vi "Launcher.vi"(8 "Globals":refnum<data-value>, 9 "E-Stop":refnum<user-event>, 10 "Response":refnum<user-event>, 11 "RequestMQ":refnum<queue>) -> ()   [LabVIEW 2020, in "Module.lvlib" / "Module.lvclass"]
doc: "This template is for the Queued Message Handler design pattern.\n\nThe Event Handling Loop generates messages based on user interface actions.\n\nThe Message Handling Loop processes messages generated by the Event Handling Loop, or by other messages. The messages are string values, so new messages can be added easily to the Message Cases case structure in the Message Handling Loop. Each message cluster can also provide an optional value for Message Data, which is a variant that can be converted to whatever message-specific data is required."
uses:
  Module.lvclass
  RPC/TypeDefs/Request.ctl
  RPC/TypeDefs/Response.ctl
  Module.lvclass/Module.ctl
  <vilib>/ErrorRing/Error Ring.xnode
  RPC.lvlib
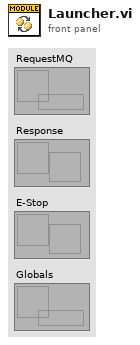
[diagram p1: front panel]
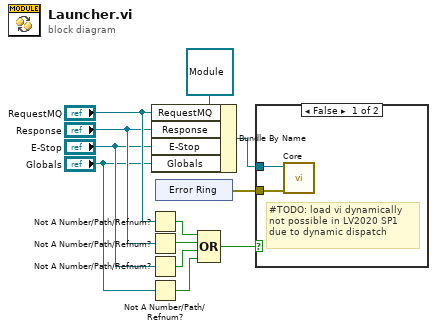
[diagram p0: block diagram]
diagram:
  n1 = Not A Number/Path/Refnum?(number/path/refnum="RequestMQ") -> (NaN/Path/Refnum?=w6:bool)
  n2 = Not A Number/Path/Refnum?(number/path/refnum="Response") -> (NaN/Path/Refnum?=w5:bool)
  n3 = Not A Number/Path/Refnum?(number/path/refnum="E-Stop") -> (NaN/Path/Refnum?=w4:bool)
  n4 = Not A Number/Path/Refnum?(number/path/refnum="Globals") -> (NaN/Path/Refnum?=w1:bool)
  n5 = Bundle By Name(cluster=refnum<class "Module.lvclass"> refnum ("Module in"), "RequestMQ"="RequestMQ", "Response"="Response", "E-Stop"="E-Stop", "Globals"="Globals") -> (w10:refnum<class "Module.lvclass">)
  n6 = xnode "Error Ring"() -> ("error out"=w12:errorcluster)
  n7 = Compound Arithmetic op=OR(w6, w5, w4, w1) -> (w3:bool)
  n8 = case shown="False" w3 {
    tunnel: w12 -> [w14 _]
    tunnel: w10 -> [w13 _]
    frame False {
      # "#TODO: load vi dynamically\nnot possible in LV2020 SP1\ndue to dynamic dispatch"
      n9 = call-dynamic "Core.vi"("error in (no error)"=w14, "Module in"=w13) -> ()  [unwired: 10 in]
    }
    frame True {
    }
  }
